vi "Set Mux.vi"(8 "error in (no error)":errorcluster, 10 "Mux Enabled Channels":bool[](array[boolean]), 11 "I2C Mux in":refnum<class "I2C MUX.lvclass">) -> (0 "error out":errorcluster, 3 "I2C Mux out":refnum<class "I2C MUX.lvclass">)   [LabVIEW 2020, in "CTI-Peripheral.lvlib" / "I2C MUX.lvclass"]
uses:
  I2C MUX.lvclass
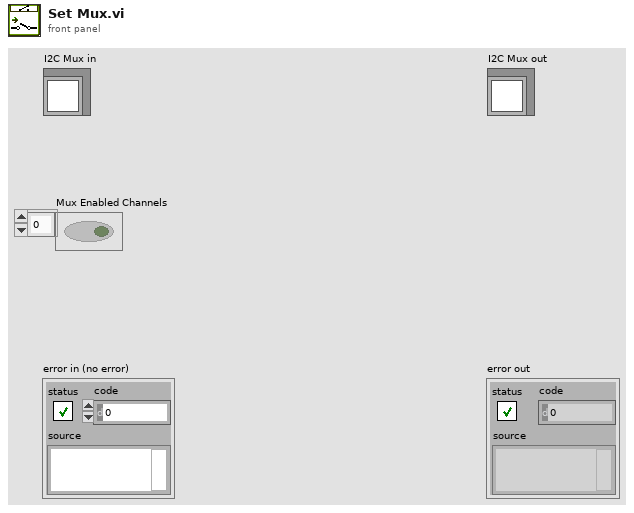
[diagram p1: front panel]
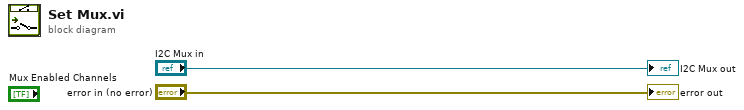
[diagram p0: block diagram]
diagram:
  "error out" <- "error in (no error)"
  "I2C Mux out" <- "I2C Mux in"
